vi "DUT Powerup.vi"() -> (0 "error out":errorcluster, 3 "Test Result":bool)   [LabVIEW 2017]
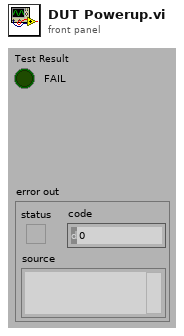
[diagram p1: front panel]
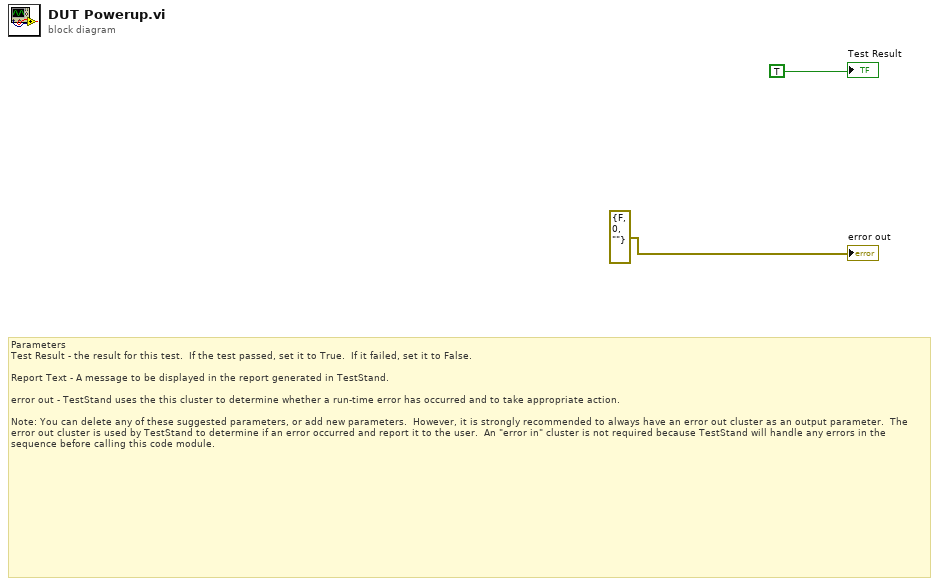
[diagram p0: block diagram]
diagram:
  # "Parameters\nTest Result - the result for this test.  If the test passed, set it to True.  If it failed, set it to False. \n\nReport Text - A message to be displayed in the report generated in TestStand. \n\nerror out - TestStand uses the this cluster to determine whether a run-time error has occurred and to take appropriate action.  \n\nNote: You can delete any of these suggested parameters, or add new parameters.  However, it is strongly recommended to always have an error out cluster as an output parameter.  The error out cluster is used by TestStand to determine if an error occurred and report it to the user.  An \"error in\" cluster is not required because TestStand will handle any errors in the sequence before calling this code module."
  "Test Result" <- TRUE
  "error out" <- errorcluster {"status"=FALSE, "code"=0, "source"=""} ("error out")
